vi "Demo.vi"() -> ()   [LabVIEW 2019]
uses:
  GLOBALS.vi
panel:
  out "size(s)":i32
  out "XY Graph":cluster{timestamp[], "Data - P":dbl[]}[](graph)
  out "error out":errorcluster
  out "Data - O2":dbl
  out "Data - P":dbl[](array[numeric])
  in  "stop":bool
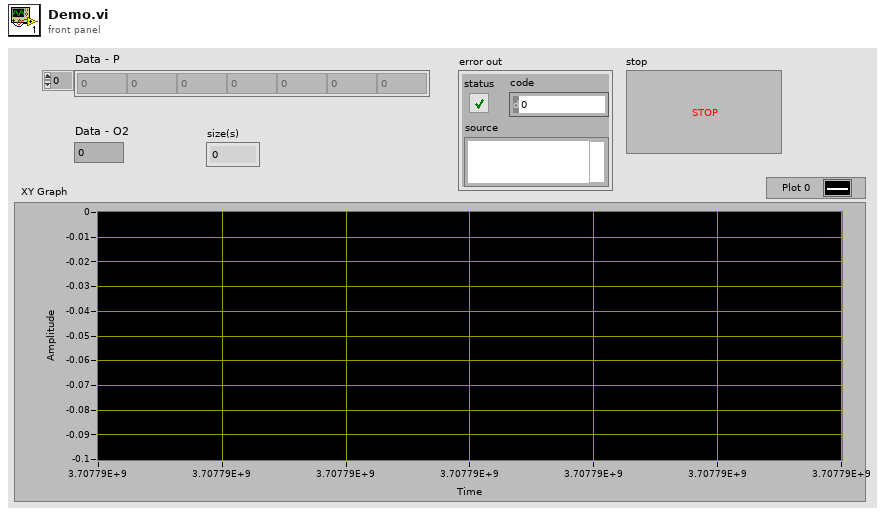
[diagram p1: front panel]
types:
  T1 = cluster{"Port":string, "Reserved By":string, "Time":timestamp}[]
  T2 = typedef "Globals_IO.ctl" = cluster{"Reserved COM ports":cluster{"Port":string, "Reserved By":string, "Time":timestamp}[]}
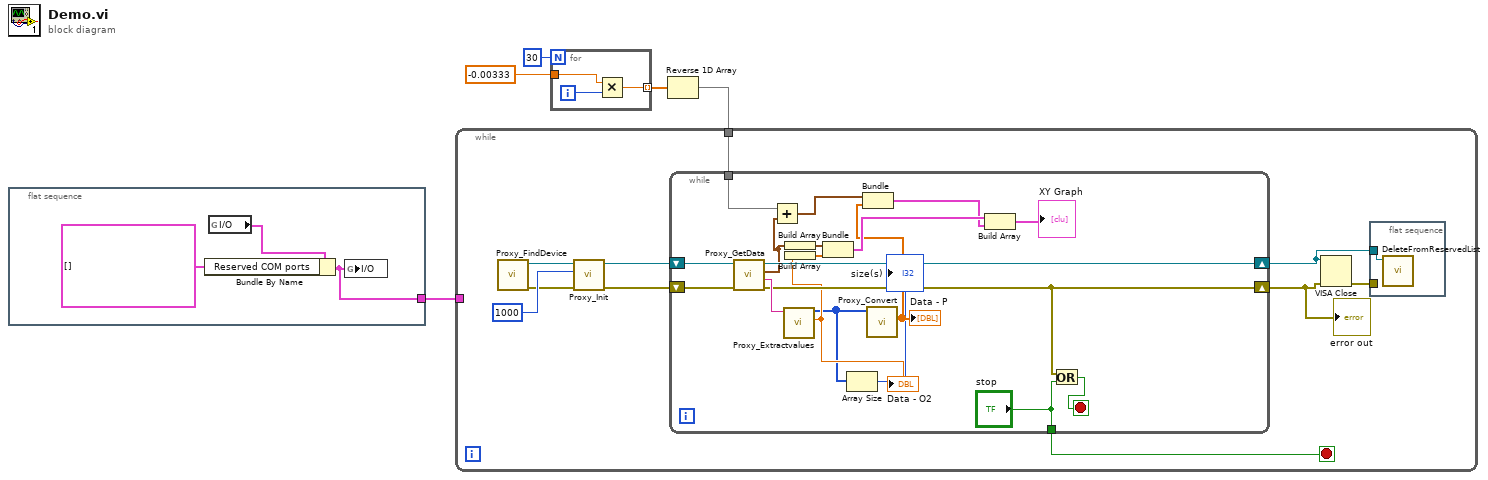
[diagram p0: block diagram]
diagram:
  n1 = flat-sequence {
    tunnel: [w6] -> w1
    frame #0 {
      n2 = global read "GLOBALS.vi" "I/O"() -> (w8:T2)
      n3 = Bundle By Name(cluster=w8, "Reserved COM ports"=T1 []) -> (w6:T2)
      n4 = global write "GLOBALS.vi" "I/O"(w6) -> ()
    }
  }
  n5 = for {
    N: 30 -> [_]
    tunnel: -0.00333 ("x") -> [w10]
    tunnel: [w9] -> w4 mode=indexing
    i -> [w11]
    n6 = Multiply(x=w10, y=w11) -> (x*y=w9:dbl)
  }
  n7 = Reverse 1D Array(array=w4) -> (reversed array=w3:dbl[])
  n8 = while {
    tunnel: w3 -> [w15]
    tunnel: w1 -> [_]
    stop <- w16 stop-if-true
    n9 = call "Proxy_FindDevice.vi"() -> ("error out"=w17:errorcluster, "VISA resource name out"=w18:refnum<visa-resource-name>)  [unwired: 10 in]
    n10 = call "Proxy_Init.vi"("error in (no error)"=w17, "Serial Options.Timeout (ms)"=1000, "VISA Refnum in"=w18) -> ("error out"=w19:errorcluster, "VISA Refnum out"=w21:refnum<visa-resource-name>)  [unwired: 7 in]
    n11 = while {
      shift-right: [w37] -> w14
      shift-left: w19 -> [w40]
      shift-right: [w38] -> w13
      shift-left: w21 -> [w41]
      tunnel: ["stop"] -> w16
      tunnel: w15 -> [w30]
      stop <- w36 stop-if-true
      n12 = call "Proxy_GetData.vi"("error in (no error)"=w40, "VISA resource name"=w41) -> ("error out"=w37:errorcluster, "Read String"=w39:string, "Time"=w29:timestamp, "VISA resource name out"=w38:refnum<visa-resource-name>)  [unwired: 6 in]
      n13 = Add(x=w30, y=w29) -> (x+y=w28:timestamp[])
      n14 = call "Proxy_Extractvalues.vi"("Read string"=w39) -> ("Data - O2"=w32:dbl, "Data - P"=w24:i16[])  [unwired: 8 in, 1 out]
      "Data - O2" <- w32
      n15 = Build Array(w29) -> (w34:timestamp[])
      n16 = Build Array(w32) -> (w33:dbl[])
      n17 = Bundle(w34, w33) -> (w31:cluster{timestamp[], dbl[]})  [unwired: 1 in]
      n18 = Array Size(array=w24) -> (size(s)=→"size(s)":i32)
      n19 = call "Proxy_Convert.vi"("Data - P"=w24) -> ("Data - P"=w27:dbl[])  [unwired: 10 in]
      "Data - P" <- w27
      n20 = Bundle(w28, "Data - P"=w27) -> (w26:cluster{timestamp[], "Data - P":dbl[]})  [unwired: 1 in]
      n21 = Build Array(w31, w26) -> (→"XY Graph":cluster{timestamp[], "Data - P":dbl[]}[])
      n22 = Or(x=w37, y="stop") -> (x .or. y?=w36:bool)
    }
    "error out" <- w14
    n23 = VISA Close(VISA resource name=w13, error in (no error)=w14) -> (error out=w12:errorcluster)
    n24 = flat-sequence {
      tunnel: w13 -> [w22]
      tunnel: w12 -> [_]
      frame #0 {
        n25 = call "DeleteFromReservedList.vi"("VISA resource"=w22) -> ()  [unwired: 10 in, 1 out]
      }
    }
  }
